vi "getXMLDetectionParameters.vi"(7 "error in":errorcluster, 10 "Detection Parameters Node":refnum<k20>) -> (0 "error out":errorcluster, 3 "Detection Parameters":T1 {"Max Intensity%" max=100 step=1})   [LabVIEW 2013]
uses:
  <vilib>/xml/NI_XML.lvlib
panel:
  out "error out 2":errorcluster
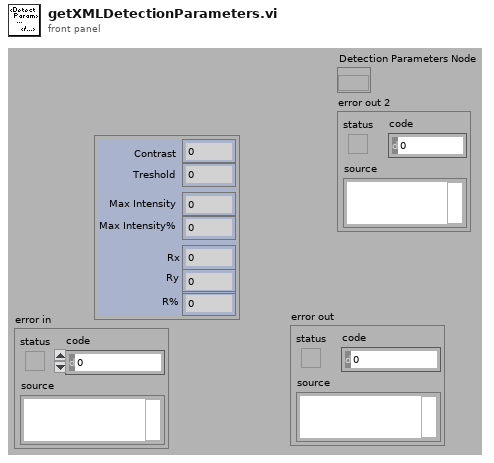
[diagram p1: front panel]
types:
  T1 = cluster{"Contrast":i32, "Treshold":u8, "Max Intensity":i32, "Max Intensity%":u8, "Rx":i32, "Ry":i32, "R%":sgl}
  T2 = cluster{"[0]":dbl, "[1]":dbl, "[2]":dbl, "[3]":dbl, "[4]":dbl, "[5]":dbl, "[6]":dbl, "[7]":dbl, "[8]":dbl}
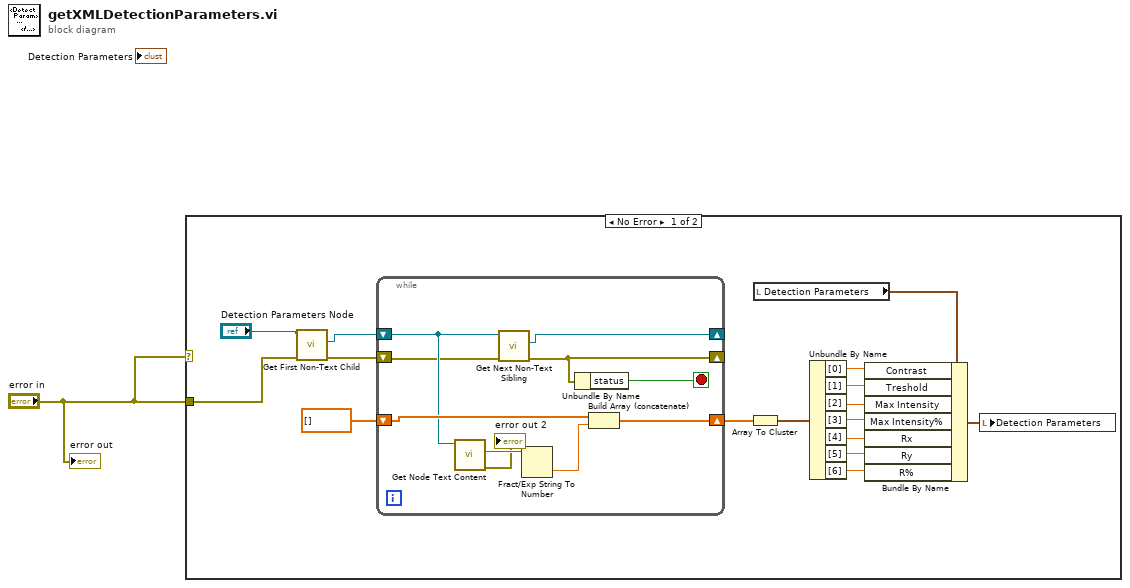
[diagram p0: block diagram]
diagram:
  n1 = case shown="No Error" "error in" {
    tunnel: "error in" -> [w4 _]
    frame No Error {
      n2 = call <vilib>:"Get First Non-Text Child.vi"("error in (no error)"=w4, "node in"="Detection Parameters Node") -> ("error out"=w3:errorcluster, "child node"=w2:refnum<k20>)  [unwired: 6 in, 2 out]
      n3 = while {
        shift-right: [w19] -> _
        shift-left: w2 -> [w22]
        shift-right: [w20] -> _
        shift-left: w3 -> [w21]
        shift-right: [w25] -> w16
        shift-left: dbl[] [] -> [w23]
        stop <- w26 stop-if-true
        n4 = call <vilib>:"Get Node Text Content.vi"("node in"=w22) -> ("error out"=→"error out 2":errorcluster, "node text"=w27:string)  [unwired: 8 in, 1 out]
        n5 = call <vilib>:"Get Next Non-Text Sibling.vi"("error in (no error)"=w21, "node in"=w22) -> ("error out"=w20:errorcluster, "sibling node"=w19:refnum<k20>)  [unwired: 6 in, 2 out]
        n6 = Fract/Exp String To Number(string=w27) -> (number=w24:dbl)  [unwired: 3 in, 1 out]
        n7 = Unbundle By Name(w20) -> ("status"=w26:bool)
        n8 = Build Array (concatenate)(w23, w24) -> (w25:dbl[])
      }
      n9 = Array To Cluster(array=w16) -> (cluster=w14:T2)
      n10 = local read "Detection Parameters"() -> (w6:T1)
      n11 = Unbundle By Name(w14) -> ("[0]"=w13:dbl, "[1]"=w12:dbl, "[2]"=w11:dbl, "[3]"=w10:dbl, "[4]"=w9:dbl, "[5]"=w8:dbl, "[6]"=w7:dbl)
      n12 = Bundle By Name(cluster=w6, "Contrast"=w13, "Treshold"=w12, "Max Intensity"=w11, "Max Intensity%"=w10, "Rx"=w9, "Ry"=w8, "R%"=w7) -> (w15:T1)
      n13 = local write "Detection Parameters"(w15) -> ()
    }
    frame Error {
    }
  }
  "error out" <- "error in"
